vi "Retract.vi"(1 "Number of Cycles":i32=10, 2 "Retracting?":bool) -> (0 "Finished?":bool)   [LabVIEW 2015]
uses:
  Globals.vi
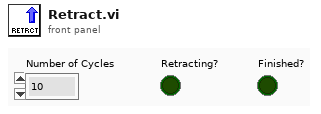
[diagram p1: front panel]
types:
  T1 = enum16{"Read XYZ Motor Position", "Read XYZ Piezo Position", "Read Setpoint", "Begin AutoLand", "Begin AutoLand, Wait till done", "XYZ Motions", "Init Scan (from global settings)", "Start Scan", "Stop Scan"}
  T2 = cluster{"Approach":bool, "Retract":bool, "Up":bool, "Up-Right":bool, "Right":bool, "Up Left":bool}
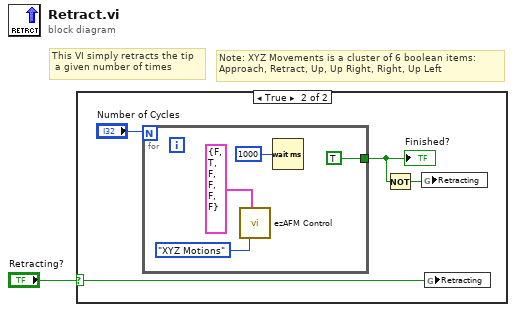
[diagram p0: block diagram]
diagram:
  # "This VI simply retracts the tip\n a given number of times"
  # "Note: XYZ Movements is a cluster of 6 boolean items: \nApproach, Retract, Up, Up Right, Right, Up Left"
  n1 = case shown="True" "Retracting?" {
    selector: "Retracting?" -> [_ w3]
    frame False {
    }
    frame True {
      n2 = for {
        N: "Number of Cycles" -> [_]
        tunnel: [TRUE] -> w2
        n3 = call "ezAFM Control.vi"("XYZ Movements"=T2 {"Approach"=FALSE, "Retract"=TRUE, "Up"=FALSE, "Up-Right"=FALSE, "Right"=FALSE, "Up Left"=FALSE}, "Mode"=T1."XYZ Motions") -> ()  [unwired: 3 in, 4 out]
        n4 = Wait (ms)(milliseconds to wait=u32 1000) -> ()  [unwired: 1 out]
      }
      "Finished?" <- w2
      n5 = Not(x=w2) -> (.not. x?=w5:bool)
      n6 = global write "Globals.vi" "Retracting"(w5) -> ()
      n7 = global write "Globals.vi" "Retracting"(w3) -> ()
    }
  }
